vi "水质.vi"(9 "Bool引用句柄":refnum<vi>, 10 "簇":T4, 11 "事件注册引用句柄":refnum<event-registration>) -> ()   [LabVIEW 2020]
uses:
  <vilib>/Utility/miscctls.llb/LVRectTypeDef.ctl
  <vilib>/Utility/miscctls.llb/LVRowAndColumnUnsignedTypeDef.ctl
  Windows/System32/user32.dll
panel:
  in  "布尔 3":T1
  in  "布尔 2":T2
  in  "布尔":T3
  out "数值":dbl format="%#_2f MΩ*cm"
  in  "表格":string[][](table)
  out "波形图":dbl[](graph)
  # "水质数据"
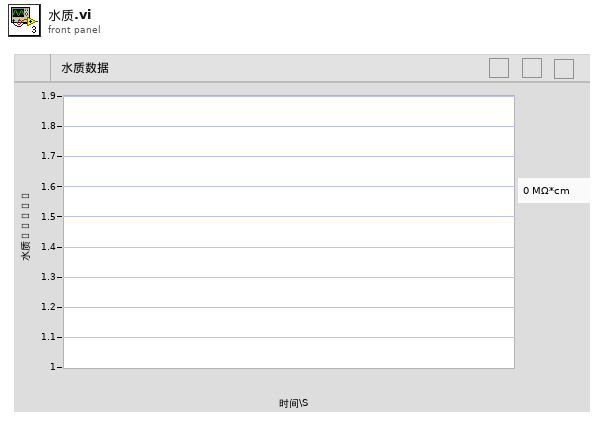
[diagram p1: front panel]
types:
  T1 = typedef "控件关闭.ctl" = bool
  T2 = typedef "控件最小化.ctl" = bool
  T3 = typedef "控件最大化.ctl" = bool
  T4 = cluster{"A1水质":refnum<vi>, "A2水质":refnum<vi>, "A3水质":refnum<vi>, "A4水质":refnum<vi>}
  T5 = typedef "LVRowAndColumnUnsignedTypeDef.ctl" = cluster{"Row":u32, "Column":u32}
  T6 = typedef "LVRectTypeDef.ctl" = cluster{"Left":i16, "Top":i16, "Right":i16, "Bottom":i16}
  T7 = typedef "LVPoint32TypeDef.ctl" = cluster{"Horizontal":i32, "Vertical":i32}
  T8 = enum32{"Invalid", "Standard", "Closed", "Hidden", "Minimized", "Maximized"}
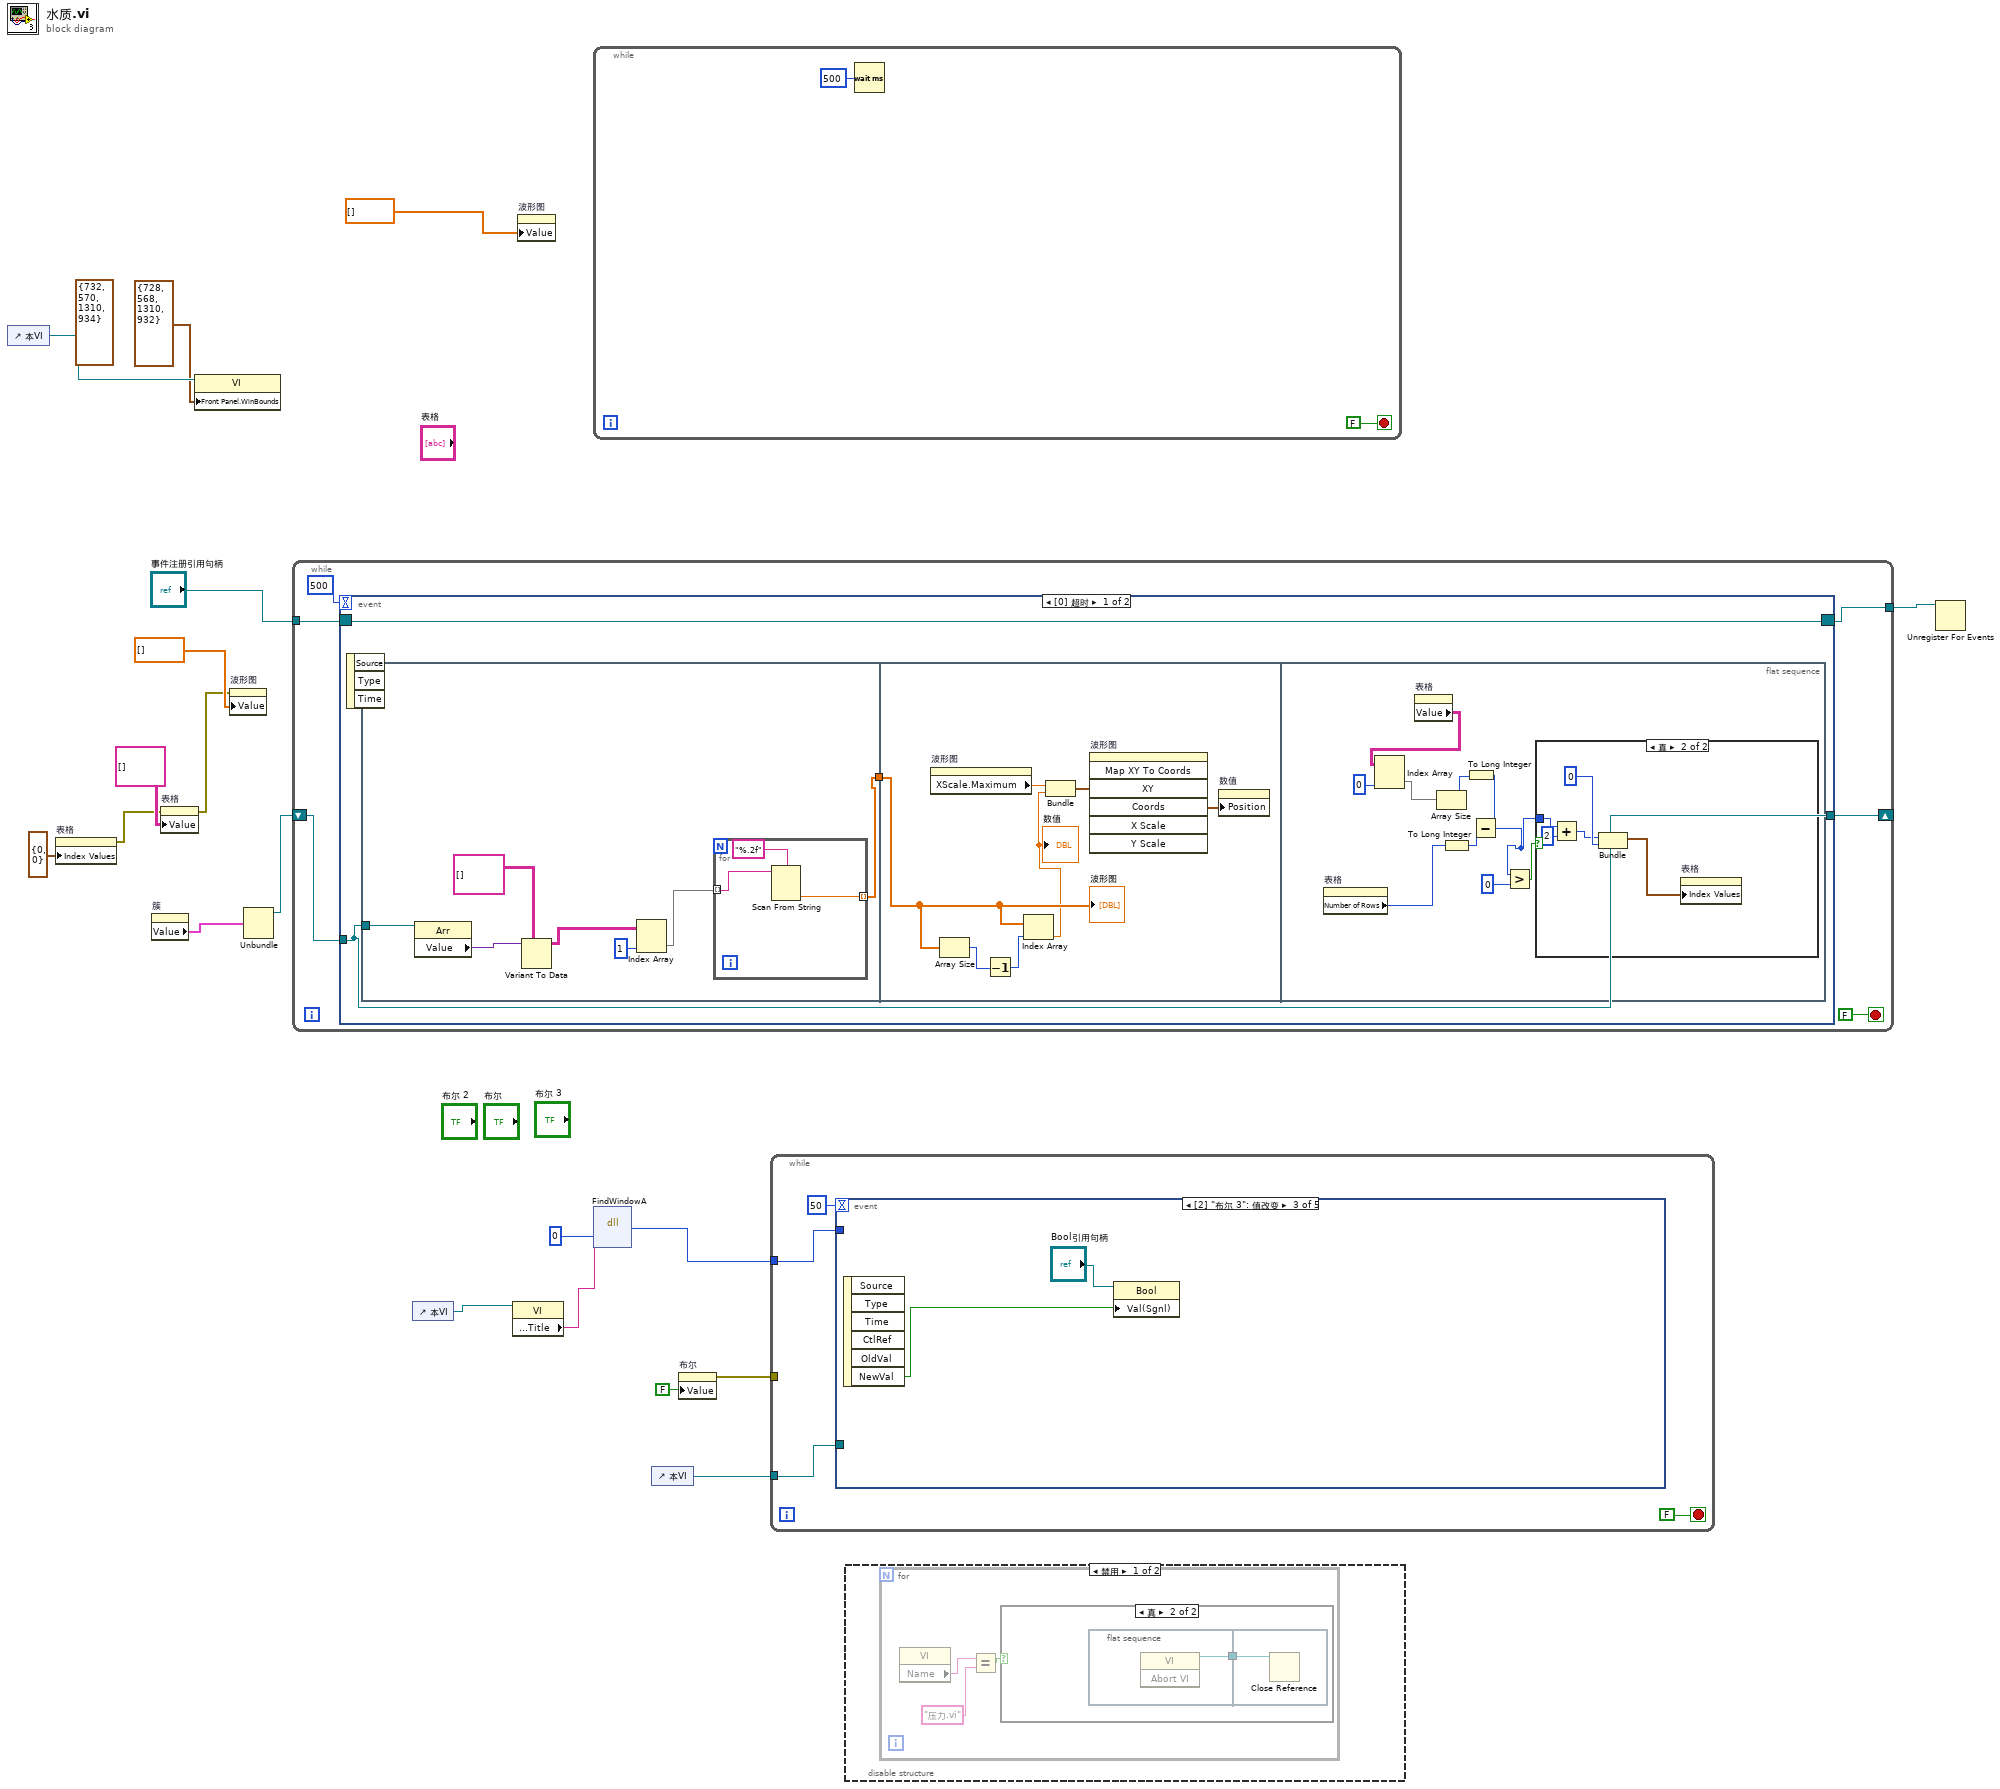
[diagram p0: block diagram]
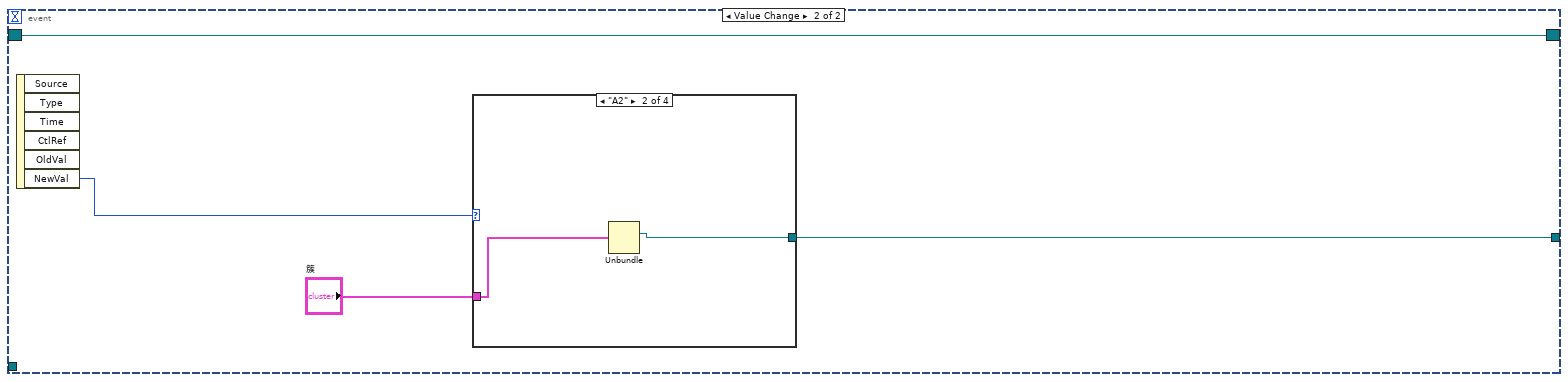
[diagram p3: hidden frame]
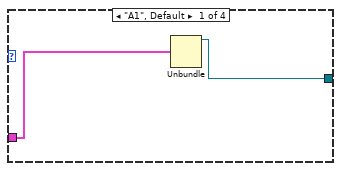
[diagram p4: hidden frame]
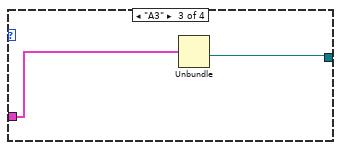
[diagram p5: hidden frame]
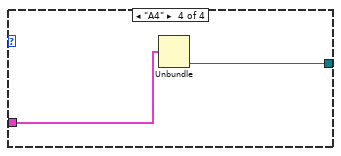
[diagram p6: hidden frame]
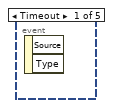
[diagram p9: hidden frame]
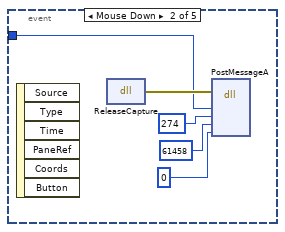
[diagram p10: hidden frame]
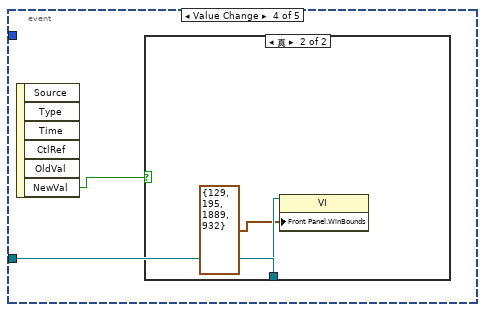
[diagram p11: hidden frame]
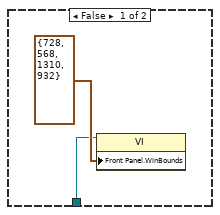
[diagram p12: hidden frame]
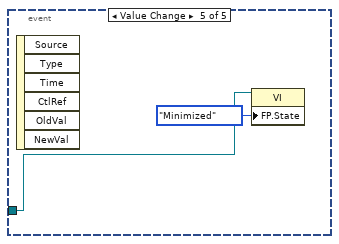
[diagram p13: hidden frame]
diagram:
  (unwired) T6 {"Left"=732, "Top"=570, "Right"=1310, "Bottom"=934} ("前面板窗口:窗口边界")
  n1 = control-ref of="本VI"() -> (w19:refnum<vi>)
  n2 = property on="表格" class="Tbl (严格)"("Index Values"=T5 {"Row"=0, "Column"=0} ("索引值")) -> (error out=w6:errorcluster)  [unwired: 2 in, 1 out]
  n3 = property on="簇" class="Clust (严格)"() -> ("Value"=w4:T4)  [unwired: 2 in, 2 out]
  n4 = property on="表格" class="Tbl (严格)"(error in=w6, "Value"=string[][] []) -> (error out=w7:errorcluster)  [unwired: 1 in, 1 out]
  n5 = property class="VI"(reference=w19, "Front Panel.WinBounds"=T6 {"Left"=728, "Top"=568, "Right"=1310, "Bottom"=932} ("前面板窗口:窗口边界")) -> ()  [unwired: 1 in, 2 out]
  n6 = property on="波形图" class="WFGraph (严格)"(error in=w7, "Value"=dbl[] []) -> ()  [unwired: 1 in, 2 out]
  n7 = Unbundle(w4) -> ("A1水质"=w3:refnum<vi>)  [unwired: 3 out]
  n8 = while {
    tunnel: "事件注册引用句柄" -> [w24]
    shift-right: [w23] -> _
    shift-left: w3 -> [w22]
    tunnel: [w21] -> w2
    stop <- FALSE stop-if-true
    n9 = event shown="[0] 超时" {
      selector: w24 -> [w28 w61]
      dyn-events: [w28 w61] -> w21
      timeout: 500 -> [_ _]
      tunnel: [w26 w62] -> w23
      tunnel: w22 -> [w26 _]
      event Timeout {
        n10 = event-data() -> ()  [unwired: 1 in, 3 out]
        n11 = flat-sequence {
          tunnel: w26 -> [w34]
          tunnel: [w30] -> w27
          tunnel: w27 -> [w41]
          frame #0 {
            n12 = property class="Arr"(reference=w34) -> ("Value"=w35:variant)  [unwired: 1 in, 2 out]
            n13 = Variant To Data(type=string[][] [], Variant=w35) -> (data=w29:string[][])  [unwired: 1 in, 1 out]
            n14 = Index Array(array=w29, index (col)=1 ("禁用的索引 (列)")) -> (element=w31:string[])  [unwired: 1 in]
            n15 = for {
              tunnel: w31 -> [w38] mode=indexing
              tunnel: [w36] -> w30 mode=indexing
              n16 = Scan From String(format string="%.2f" ("格式字符串"), input string=w38) -> (output 1=w36:dbl)  [unwired: 3 in, 3 out]
            }
          }
          frame #1 {
            n17 = property on="波形图" class="WFGraph (严格)"() -> ("XScale.Maximum"=w43:dbl)  [unwired: 2 in, 2 out]
            n18 = Array Size(array=w41) -> (size(s)=w42:i32)
            n19 = Decrement(x=w42) -> (x-1=w40:i32)
            n20 = Index Array(array=w41, index=w40) -> (element=w39:dbl)
            "数值" <- w39
            n21 = Bundle("XScale.Maximum"=w43, w39) -> (w44:cluster{"XScale.Maximum":dbl, dbl})  [unwired: 1 in]
            n22 = invoke on="波形图" class="WFGraph (严格)" method="Map XY To Coords"("XY"=w44) -> ("Coords"=w45:T7)  [unwired: 6 in, 6 out]
            n23 = property on="数值" class="DigNum (严格)"("Position"=w45) -> ()  [unwired: 2 in, 2 out]
            "波形图" <- w41
          }
          frame #2 {
            n24 = property on="表格" class="Tbl (严格)"() -> ("Number of Rows"=w47:u32)  [unwired: 2 in, 2 out]
            n25 = property on="表格" class="Tbl (严格)"() -> ("Value"=w46:string[][])  [unwired: 2 in, 2 out]
            n26 = Index Array(array=w46, index (col)=0 ("禁用的索引 (列)")) -> (element=w54:string[])  [unwired: 1 in]
            n27 = Array Size(array=w54) -> (size(s)=w52:i32)
            n28 = To Long Integer(number=w47) -> (32bit integer=w50:i32)
            n29 = To Long Integer(number=w52) -> (32bit integer=w51:i32)
            n30 = Subtract(x=w51, y=w50) -> (x-y=w48:i32)
            n31 = Greater?(x=w48, y=0) -> (0:w53:bool)
            n32 = case shown="真" w53 {
              tunnel: w48 -> [_ w59]
              frame False {
              }
              frame True {
                n33 = Add(x=w59, y=2) -> (x+y=w57:i32)
                n34 = Bundle(w57, 0) -> (w56:cluster{i32, i32})  [unwired: 1 in]
                n35 = property on="表格" class="Tbl (严格)"("Index Values"=w56) -> ()  [unwired: 2 in, 2 out]
              }
            }
          }
        }
      }
      event Value Change {
        n36 = event-data() -> ("NewVal"=w64:enum32{"未选择", "A1", "A2", "A3", "A4"})  [unwired: 1 in, 5 out]
        n37 = case shown="\"A2\"" w64 {
          tunnel: "簇" -> [w66 w68 w70 w72]
          tunnel: [w65 w67 w69 w71] -> w62
          frame "A1", Default {
            n38 = Unbundle(w66) -> ("A1水质"=w65:refnum<vi>)  [unwired: 3 out]
          }
          frame "A2" {
            n39 = Unbundle(w68) -> ("A2水质"=w67:refnum<vi>)  [unwired: 3 out]
          }
          frame "A3" {
            n40 = Unbundle(w70) -> ("A3水质"=w69:refnum<vi>)  [unwired: 3 out]
          }
          frame "A4" {
            n41 = Unbundle(w72) -> ("A4水质"=w71:refnum<vi>)  [unwired: 3 out]
          }
        }
      }
    }
  }
  n42 = control-ref of="本VI"() -> (w17:refnum<vi>)
  n43 = property class="VI"(reference=w17) -> ("Front Panel.Title"=w16:string)  [unwired: 1 in, 2 out]
  n44 = property on="波形图" class="WFGraph (严格)"("Value"=dbl[] [] ("波形图")) -> ()  [unwired: 2 in, 2 out]
  n45 = while {
    stop <- FALSE stop-if-true
    n46 = Wait (ms)(milliseconds to wait=u32 500 ("等待时间（毫秒）")) -> ()  [unwired: 1 out]
  }
  n47 = dll-call lib="/Windows/System32/user32.dll" fn="FindWindowA"("lp"=u32 0, "name"=w16) -> ("返回类型"=w15:u32)  [unwired: 5 in, 2 out]
  n48 = control-ref of="本VI"() -> (w11:refnum<vi>)
  n49 = property on="布尔" class="Bool (严格)"("Value"=T3 FALSE ("布尔")) -> (error out=w12:errorcluster)  [unwired: 2 in, 1 out]
  n50 = while {
    tunnel: w15 -> [w78]
    tunnel: w12 -> [_]
    tunnel: w11 -> [w77]
    stop <- FALSE stop-if-true
    n51 = event shown="[2] \"布尔 3\": 值改变" {
      selector: _ -> [_ _ _ _ _]
      dyn-events: _ -> [_ _ _ _ _]
      timeout: 50 -> [_ _ _ _ _]
      tunnel: w78 -> [_ w82 _ _ _]
      tunnel: w77 -> [_ _ _ w86 w93]
      event Timeout {
        n52 = event-data() -> ()  [unwired: 1 in, 2 out]
      }
      event Mouse Down {
        n53 = event-data() -> ()  [unwired: 1 in, 6 out]
        n54 = dll-call lib="/Windows/System32/user32.dll" fn="ReleaseCapture"() -> (error out=w83:errorcluster)  [unwired: 4 in, 1 out]
        n55 = dll-call lib="/Windows/System32/user32.dll" fn="PostMessageA"(error in=w83, "lp"=w82, "name"=274, "vak"=61458, "val"=0) -> ()  [unwired: 7 in, 2 out]
      }
      event Value Change {
        n56 = event-data() -> ("NewVal"=w85:T1)  [unwired: 1 in, 5 out]
        n57 = property class="Bool"(reference="Bool引用句柄", "Val(Sgnl)"=w85) -> ()  [unwired: 1 in, 2 out]
      }
      event Value Change {
        n58 = event-data() -> ("NewVal"=w87:T3)  [unwired: 1 in, 5 out]
        n59 = case shown="真" w87 {
          tunnel: w86 -> [w88 w91]
          frame False {
            n60 = property class="VI"(reference=w88, "Front Panel.WinBounds"=T6 {"Left"=728, "Top"=568, "Right"=1310, "Bottom"=932} ("前面板窗口:窗口边界")) -> ()  [unwired: 1 in, 2 out]
          }
          frame True {
            n61 = property class="VI"(reference=w91, "Front Panel.WinBounds"=T6 {"Left"=129, "Top"=195, "Right"=1889, "Bottom"=932} ("前面板窗口:前面板边界")) -> ()  [unwired: 1 in, 2 out]
          }
        }
      }
      event Value Change {
        n62 = event-data() -> ()  [unwired: 1 in, 6 out]
        n63 = property class="VI"(reference=w93, "FP.State"=T8."Minimized" ("前面板窗口:状态")) -> ()  [unwired: 1 in, 2 out]
      }
    }
  }
  n64 = disable-structure shown="禁用" {
    frame Disabled {
      n65 = for {
        n66 = property class="VI"() -> ("Name"=w96:string)  [unwired: 2 in, 2 out]
        n67 = Equal?(x=w96, y="压力.vi") -> (x = y?=w94:bool)
        n68 = case shown="真" w94 {
          frame False {
          }
          frame True {
            n69 = flat-sequence {
              tunnel: [w98] -> w97
              tunnel: w97 -> [w99]
              frame #0 {
                n70 = invoke class="VI" method="Abort VI"() -> (reference out=w98:refnum<vi>)  [unwired: 3 in, 2 out]
              }
              frame #1 {
                n71 = Close Reference(reference=w99) -> ()  [unwired: 1 in, 1 out]
              }
            }
          }
        }
      }
    }
    frame Enabled {
    }
  }
  n72 = Unregister For Events(event registration refnum=w2) -> ()  [unwired: 1 in, 1 out]
